vi "Cache.Init.vi"(8 "error in (no error)":errorcluster, 10 "VariantsInUse":string[](array[string])) -> (0 "error out":errorcluster)   [LabVIEW 2016]
uses:
  Cache.SystemID.Fglb.Action.ctl
  Cache.TestSteps.Fglb.Action.ctl
  Cache.Status.Fglb.Action.ctl
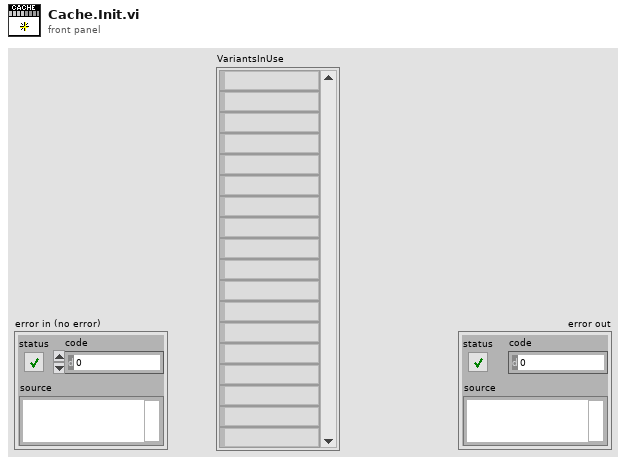
[diagram p1: front panel]
types:
  T1 = typedef "Cache.Status.Fglb.Action.ctl" = enum16{"init", "Changeover", "CheckStatus", "NewData", "get"}
  T2 = typedef "Cache.TestSteps.Fglb.Action.ctl" = enum16{"init", "add", "get"}
  T3 = typedef "Cache.SystemID.Fglb.Action.ctl" = enum16{"init", "add", "get"}
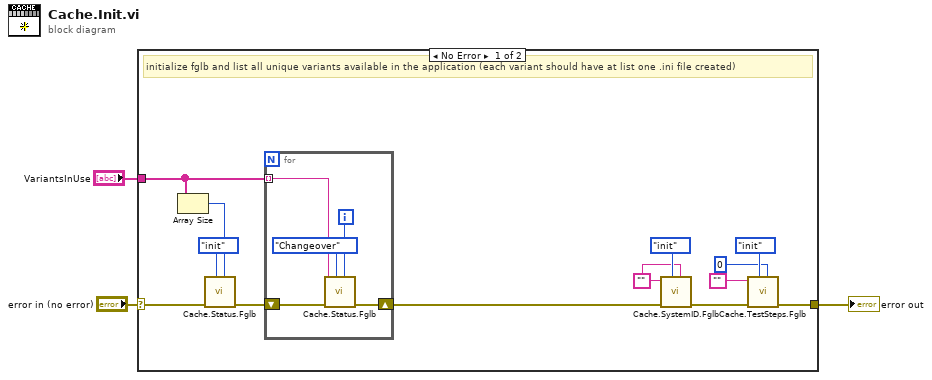
[diagram p0: block diagram]
diagram:
  n1 = case shown="No Error" "error in (no error)" {
    selector: "error in (no error)" -> [w9 w22]
    tunnel: [w13 w22] -> w3
    tunnel: "VariantsInUse" -> [w6 _]
    frame No Error {
      w12 = ""
      # "initialize fglb and list all unique variants available in the application (each variant should have at list one .ini file created)"
      n2 = Array Size(array=w6) -> (size(s)=w5:i32)
      n3 = call "Cache.Status.Fglb.vi"("SystemIdx"=w5, "Action (get)"=Cache.Status.Fglb.Action."init", "error in (no error)"=w9) -> ("error out"=w7:errorcluster)  [unwired: 7 in, 1 out]
      n4 = for {
        tunnel: w6 -> [w18] mode=indexing
        shift-right: [w19] -> w4
        shift-left: w7 -> [w20]
        i -> [w17]
        n5 = call "Cache.Status.Fglb.vi"("SystemIdx"=w17, "Action (get)"=Cache.Status.Fglb.Action."Changeover", "error in (no error)"=w20, "Changeover"=w18) -> ("error out"=w19:errorcluster)  [unwired: 6 in, 1 out]
      }
      n6 = call "Cache.SystemID.Fglb.vi"("Station"=w12, "Action (get)"=Cache.SystemID.Fglb.Action."init", "error in (no error)"=w4, "Variant"=w12) -> ("error out"=w16:errorcluster)  [unwired: 5 in, 2 out]
      n7 = call "Cache.TestSteps.Fglb.vi"("SystemIdx"=0, "Action (get)"=Cache.TestSteps.Fglb.Action."init", "error in (no error)"=w16, "Variant"="") -> ("error out"=w13:errorcluster)  [unwired: 4 in, 3 out]
    }
    frame Error {
    }
  }
  "error out" <- w3
